vi "i q sum 16spc.vi"(9 "input valid":bool=TRUE, 10 "IQ in 2":T1[](array[typedef])=[{"I"=0.0, "Q"=0.0, "overflow"=FALSE}, {"I"=0.0, "Q"=0.0, "overflow"=FALSE}, {"I"=0.0, "Q"=0.0, "overflow"=FALSE}, {"I"=0.0, "Q"=0.0, "overflow"=FALSE}, {"I"=0.0, "Q"=0.0, "overflow"=FALSE}, {"I"=0.0, "Q"=0.0, "overflow"=FALSE}, {"I"=0.0, "Q"=0.0, "overflow"=FALSE}, {"I"=0.0, "Q"=0.0, "overflow"=FALSE}, {"I"=0.0, "Q"=0.0, "overflow"=FALSE}, {"I"=0.0, "Q"=0.0, "overflow"=FALSE}, {"I"=0.0, "Q"=0.0, "overflow"=FALSE}, {"I"=0.0, "Q"=0.0, "overflow"=FALSE}, {"I"=0.0, "Q"=0.0, "overflow"=FALSE}, {"I"=0.0, "Q"=0.0, "overflow"=FALSE}, {"I"=0.0, "Q"=0.0, "overflow"=FALSE}, {"I"=0.0, "Q"=0.0, "overflow"=FALSE}], 11 "IQ in":T1[](array[typedef])=[{"I"=0.0, "Q"=0.0, "overflow"=FALSE}, {"I"=0.0, "Q"=0.0, "overflow"=FALSE}, {"I"=0.0, "Q"=0.0, "overflow"=FALSE}, {"I"=0.0, "Q"=0.0, "overflow"=FALSE}, {"I"=0.0, "Q"=0.0, "overflow"=FALSE}, {"I"=0.0, "Q"=0.0, "overflow"=FALSE}, {"I"=0.0, "Q"=0.0, "overflow"=FALSE}, {"I"=0.0, "Q"=0.0, "overflow"=FALSE}, {"I"=0.0, "Q"=0.0, "overflow"=FALSE}, {"I"=0.0, "Q"=0.0, "overflow"=FALSE}, {"I"=0.0, "Q"=0.0, "overflow"=FALSE}, {"I"=0.0, "Q"=0.0, "overflow"=FALSE}, {"I"=0.0, "Q"=0.0, "overflow"=FALSE}, {"I"=0.0, "Q"=0.0, "overflow"=FALSE}, {"I"=0.0, "Q"=0.0, "overflow"=FALSE}, {"I"=0.0, "Q"=0.0, "overflow"=FALSE}]) -> (2 "output valid":bool, 3 "IQ out":T1[](array[typedef]))   [LabVIEW 2021]
doc: "sum 2 IQ datas (I+I =>I ; Q+Q =>Q ; overflow or overflow or +overflow => overflow"
uses:
  <instrlib>/_niInstr/DSP/v1/Shared/Public/IQ Data.ctl
  <instrlib>/_niInstr/DSP/v1/Shared/niInstr DSP v1 Shared.lvlib
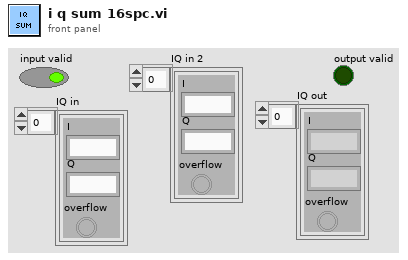
[diagram p1: front panel]
types:
  T1 = typedef "niInstr DSP v1 Shared.lvlib/IQ Data.ctl" = cluster{"I":fxp<+/-,18,1>, "Q":fxp<+/-,18,1>, "overflow":bool}
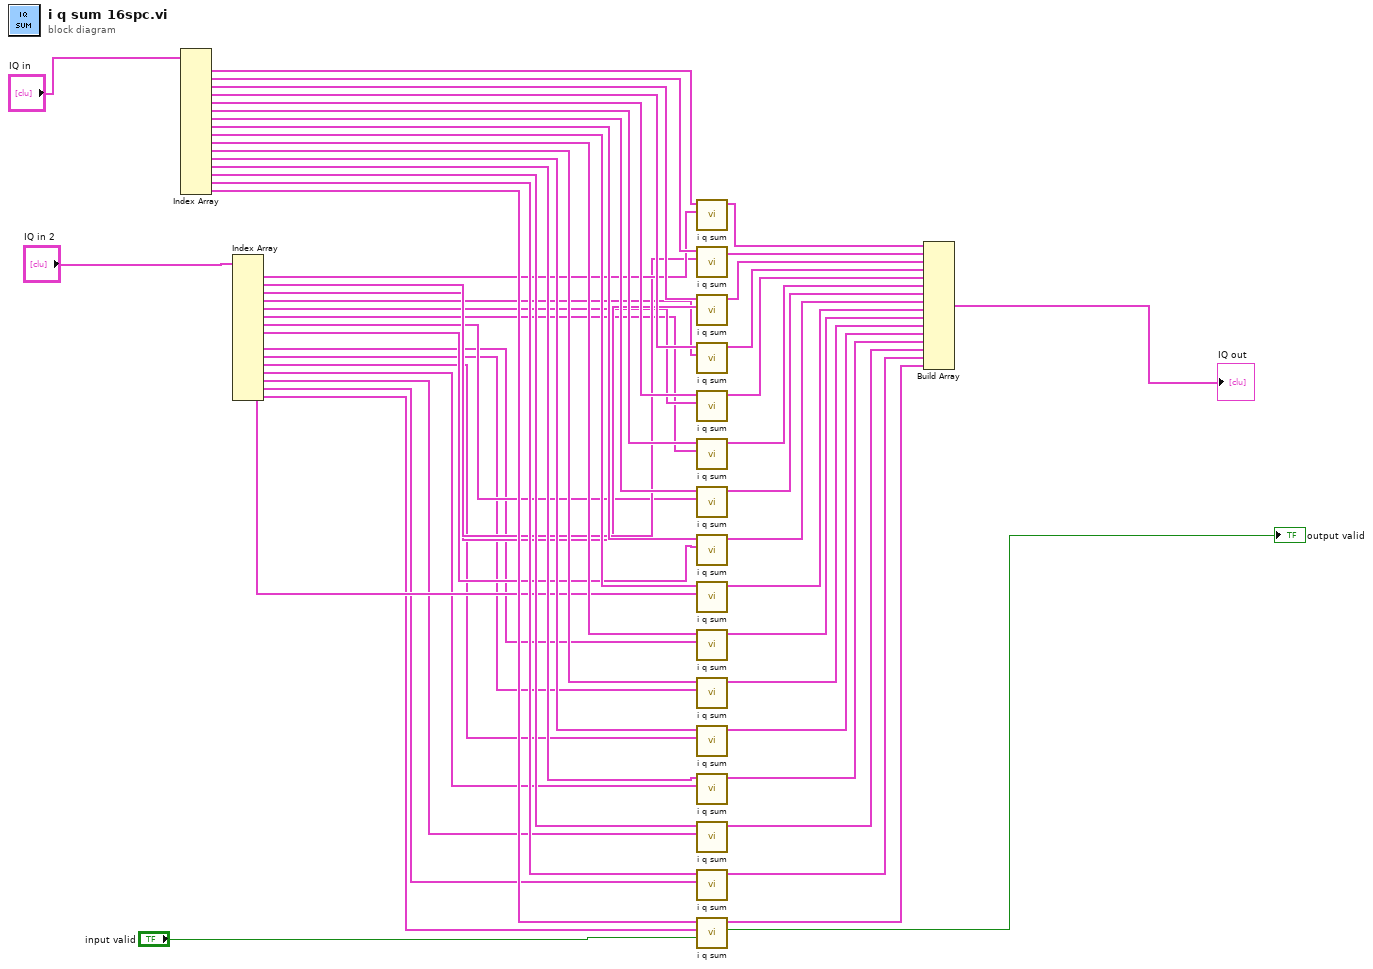
[diagram p0: block diagram]
diagram:
  n1 = Index Array(array="IQ in") -> (element #1=w51:T1, element #2=w50:T1, element #3=w49:T1, element #4=w48:T1, element #5=w47:T1, element #6=w46:T1, element #7=w45:T1, element #8=w44:T1, element #9=w43:T1, element #10=w42:T1, element #11=w41:T1, element #12=w40:T1, element #13=w39:T1, element #14=w38:T1, element #15=w37:T1, element #16=w36:T1)  [unwired: 16 in]
  n2 = Index Array(array="IQ in 2") -> (element #1=w35:T1, element #2=w34:T1, element #3=w33:T1, element #4=w32:T1, element #5=w31:T1, element #6=w30:T1, element #7=w29:T1, element #8=w28:T1, element #9=w27:T1, element #10=w26:T1, element #11=w25:T1, element #12=w24:T1, element #13=w23:T1, element #14=w22:T1, element #15=w21:T1, element #16=w20:T1)  [unwired: 16 in]
  n3 = call "i q sum.vi"(10:"data in"=w35, 11:"data in"=w51) -> ("output cluster"=w18:T1)  [unwired: 8 in, 1 out]
  n4 = call "i q sum.vi"(10:"data in"=w34, 11:"data in"=w50) -> ("output cluster"=w17:T1)  [unwired: 8 in, 1 out]
  n5 = call "i q sum.vi"(10:"data in"=w33, 11:"data in"=w49) -> ("output cluster"=w16:T1)  [unwired: 8 in, 1 out]
  n6 = call "i q sum.vi"(10:"data in"=w32, 11:"data in"=w48) -> ("output cluster"=w15:T1)  [unwired: 8 in, 1 out]
  n7 = call "i q sum.vi"(10:"data in"=w31, 11:"data in"=w47) -> ("output cluster"=w14:T1)  [unwired: 8 in, 1 out]
  n8 = call "i q sum.vi"(10:"data in"=w30, 11:"data in"=w46) -> ("output cluster"=w13:T1)  [unwired: 8 in, 1 out]
  n9 = call "i q sum.vi"(10:"data in"=w29, 11:"data in"=w45) -> ("output cluster"=w12:T1)  [unwired: 8 in, 1 out]
  n10 = call "i q sum.vi"(10:"data in"=w28, 11:"data in"=w44) -> ("output cluster"=w11:T1)  [unwired: 8 in, 1 out]
  n11 = call "i q sum.vi"(10:"data in"=w27, 11:"data in"=w43) -> ("output cluster"=w10:T1)  [unwired: 8 in, 1 out]
  n12 = call "i q sum.vi"(10:"data in"=w26, 11:"data in"=w42) -> ("output cluster"=w9:T1)  [unwired: 8 in, 1 out]
  n13 = call "i q sum.vi"(10:"data in"=w25, 11:"data in"=w41) -> ("output cluster"=w8:T1)  [unwired: 8 in, 1 out]
  n14 = call "i q sum.vi"(10:"data in"=w24, 11:"data in"=w40) -> ("output cluster"=w7:T1)  [unwired: 8 in, 1 out]
  n15 = call "i q sum.vi"(10:"data in"=w23, 11:"data in"=w39) -> ("output cluster"=w6:T1)  [unwired: 8 in, 1 out]
  n16 = call "i q sum.vi"(10:"data in"=w22, 11:"data in"=w38) -> ("output cluster"=w5:T1)  [unwired: 8 in, 1 out]
  n17 = call "i q sum.vi"(10:"data in"=w21, 11:"data in"=w37) -> ("output cluster"=w4:T1)  [unwired: 8 in, 1 out]
  n18 = call "i q sum.vi"("input valid"="input valid", 10:"data in"=w20, 11:"data in"=w36) -> ("output valid"=→"output valid":bool, "output cluster"=w3:T1)  [unwired: 7 in]
  n19 = Build Array(w18, w17, w16, w15, w14, w13, w12, w11, w10, w9, w8, w7, w6, w5, w4, w3) -> (→"IQ out":T1[])
